vi "Determine if Running in Debug Mode.vi"(9 "App.Args":string[](array[string]), 10 "App.Kind":T1(ring), 11 "Launcher VI ref":refnum<vi>) -> (2 "Debug mode?":bool)   [LabVIEW 2020, in "Launcher Support.lvlib"]
doc: "The launcher VI is meant to be run as a headless launcher for the module main VI. The launcher VI can be used as a debugging tool.\n\nThis VI determines if the launcher VI is running as a debugger by parsing the command line arguments or checking if the VI is running in development mode and sets the Launcher VI properties accordingly.\n_____\nBased on DQMH Project Template 6.1.0.94."
uses:
  Launcher Support.lvlib
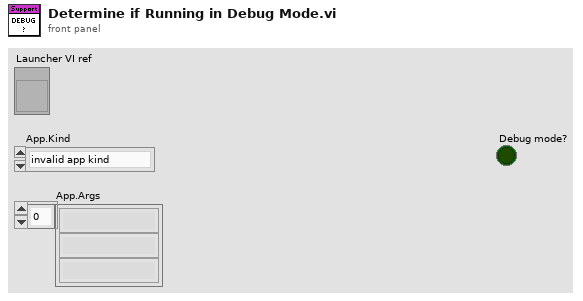
[diagram p1: front panel]
types:
  T1 = enum32{"invalid app kind", "Development System", "Run Time System", "Student Edition", "Embedded LabVIEW", "Evaluation", "Custom"}
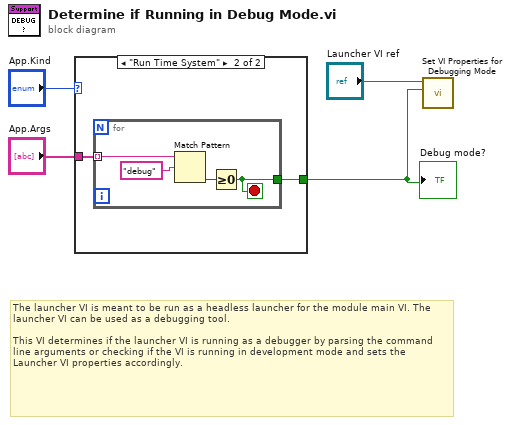
[diagram p0: block diagram]
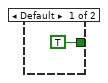
[diagram p2: hidden frame]
diagram:
  # "The launcher VI is meant to be run as a headless launcher for the module main VI. The launcher VI can be used as a debugging tool.\n\nThis VI determines if the launcher VI is running as a debugger by parsing the command line arguments or checking if the VI is running in development mode and sets the Launcher VI properties accordingly."
  n1 = case shown="\"Run Time System\"" "App.Kind" {
    tunnel: "App.Args" -> [_ w7]
    tunnel: [TRUE w6] -> w4
    frame Default {
    }
    frame "Run Time System" {
      n2 = for {
        tunnel: w7 -> [w11] mode=indexing
        tunnel: [w8] -> w6
        stop <- w8 stop-if-true
        n3 = Match Pattern(string=w11, regular expression="debug") -> (offset past match=w9:i32)  [unwired: 1 in, 3 out]
        n4 = Greater Or Equal To 0?(x=w9) -> (x >= 0?=w8:bool)
      }
    }
  }
  "Debug mode?" <- w4
  n5 = call "Set VI Properties for Debugging Mode.vi"("Debug mode?"=w4, "Launcher VI ref"="Launcher VI ref") -> ()  [unwired: 8 in, 2 out]
